vi "Even.vi"(7 "Even":bool, 11 "Array In":dbl[][](array[numeric])) -> (3 "Array Out":dbl[][](array[numeric]))   [LabVIEW 2018]
panel:
  out "x/y":dbl
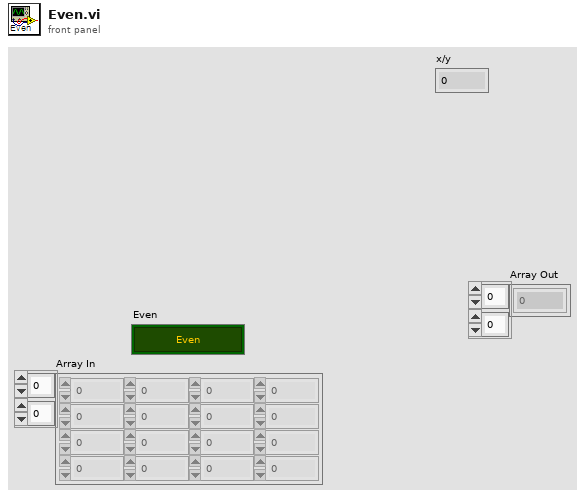
[diagram p1: front panel]
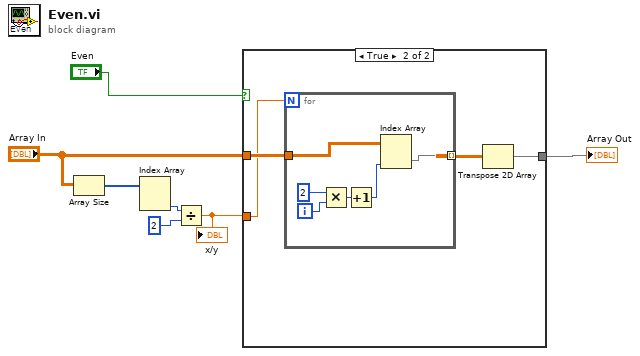
[diagram p0: block diagram]
diagram:
  n1 = Array Size(array="Array In") -> (size(s)=w6:i32[])
  n2 = Index Array(array=w6) -> (element #2=w4:i32)  [unwired: 2 in, 1 out]
  n3 = Divide(x=w4, y=2) -> (x/y=w1:dbl)
  "x/y" <- w1
  n4 = case shown="True" "Even" {
    tunnel: [w8 w9] -> w3
    tunnel: "Array In" -> [w8 w11]
    tunnel: w1 -> [_ w10]
    frame False {
    }
    frame True {
      n5 = for {
        N: w10 -> [_]
        tunnel: [w17] -> w12 mode=indexing
        tunnel: w11 -> [w18]
        i -> [w16]
        n6 = Multiply(x=2, y=w16) -> (x*y=w14:i32)
        n7 = Increment(x=w14) -> (x+1=w13:i32)
        n8 = Index Array(array=w18, index (col)=w13) -> (element=w17:dbl[])  [unwired: 1 in]
      }
      n9 = Transpose 2D Array(2D array=w12) -> (transposed array=w9:dbl[][])
    }
  }
  "Array Out" <- w3
